vi "New.vi"(7 "position":T1=10 items=["Open"=10, "Closed"=11], 8 "error in (no error)":errorcluster, 9 "property":refnum<k21>, 10 "physical channel name":refnum<k21>="$DefaultPhysChans", 11 "Name":string) -> (0 "error out":errorcluster, 3 "PhysicalChannelRelay out":refnum<class "PhysicalChannelRelay.lvclass">)   [LabVIEW 2015, in "PhysicalChannelRelay.lvclass"]
doc: "This creates a new RelayInterface object for control via a physical channel and/or command."
uses:
  PhysicalChannelRelay.lvclass
  slscsl/RelayPosition.ctl
  PhysicalChannelRelay.lvclass/PhysicalChannelRelay.ctl
  Relay Interface/RelayInterface.lvclass
  slscsl/slscsl.lvclass
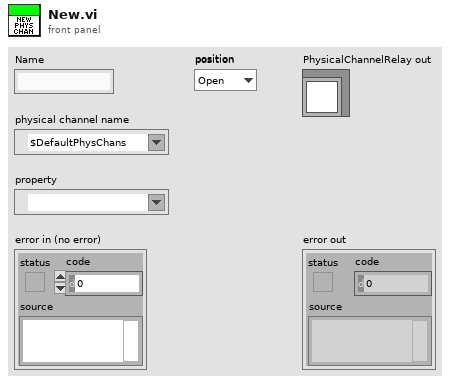
[diagram p1: front panel]
types:
  T1 = typedef "slscsl.lvclass/RelayPosition.ctl" = i32
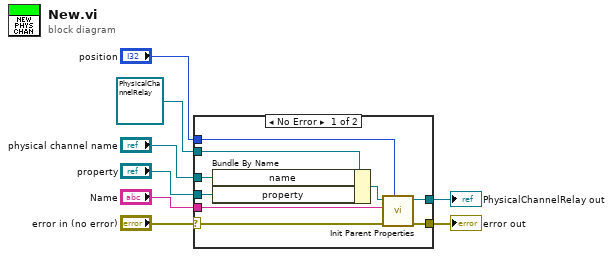
[diagram p0: block diagram]
diagram:
  n1 = case shown="No Error" "error in (no error)" {
    selector: "error in (no error)" -> [w11 w19]
    tunnel: [w12 w19] -> w7
    tunnel: [w13 w18] -> w5
    tunnel: refnum<class "PhysicalChannelRelay.lvclass"> refnum ("PhysicalChannelRelay in") -> [w17 w18]
    tunnel: "physical channel name" -> [w16 _]
    tunnel: "property" -> [w15 _]
    tunnel: "Name" -> [w10 _]
    tunnel: "position" -> [w9 _]
    frame No Error {
      n2 = Bundle By Name(cluster=w17, "name"=w16, "property"=w15) -> (w14:refnum<class "PhysicalChannelRelay.lvclass">)
      n3 = call "Init Parent Properties.vi"("position"=w9, "error in (no error)"=w11, "Name"=w10, "RelayInterface in"=w14) -> ("error out"=w12:errorcluster, "RelayInterface out"=w13:refnum<class "PhysicalChannelRelay.lvclass">)  [unwired: 6 in]
    }
    frame Error {
    }
  }
  "error out" <- w7
  "PhysicalChannelRelay out" <- w5
